vi "Measure.vi"(8 "error in":errorcluster, 10 "Measure Type":i32(ring) items=["Current", "High Current", "Low Current", "Max Current", "Min Current", "Power", "Voltage", "High Voltage", "Low Voltage", "Max Voltage", "Min Voltage", "A Hour", "W Hour", "Local Voltage", "Remote Voltage", "V/I/P/AHour/WHour", "Original Current", "Original Voltage", "UI interface Meter current", "UI Meter Voltage", "UI Meter power"], 11 "VISA resource name":refnum<visa-resource-name>) -> (0 "error out":errorcluster, 2 "Value":string, 3 "VISA resource name out":refnum<visa-resource-name>)   [LabVIEW 2015, in "IT-M3900C.lvlib"]
doc: "The MEASure subsystem command measures the output voltage or current.These commands will trigger the acquisition of additional data before the readings are returned.Perform the measurement by digitizing the instantaneous output voltage or current at the specified measurement time, storing the result in the buffer and calculating the value of the specified measurement type.\n\n<b>Measure Type</b>\n0:Current\n1:High Current\n2:Low Current\n3:Max Current\n4:Min Current\n5:Power\n6:Voltage\n7:High Voltage\n8:Low Voltage\n9:Max Voltage\n10:Min Voltage\n11:A Hour\n12:W Hour\n13:Local Voltage\n14:Remote Voltage\n15:V/I/P/AHour/WHour\n16:Original Current\n17:Original Voltage\n18:UI Meter current\n19:UI Meter voltage\n20:UI Meter power"
uses:
  <instrlib>/IT-M3900C/IT-M3900C.lvlib
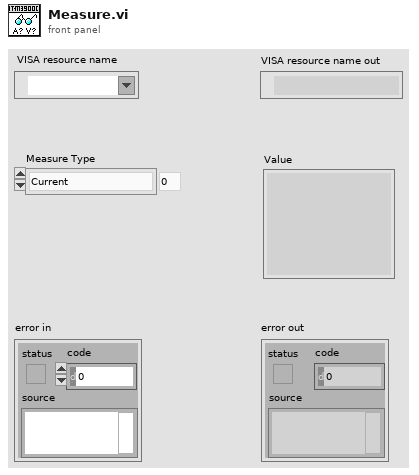
[diagram p1: front panel]
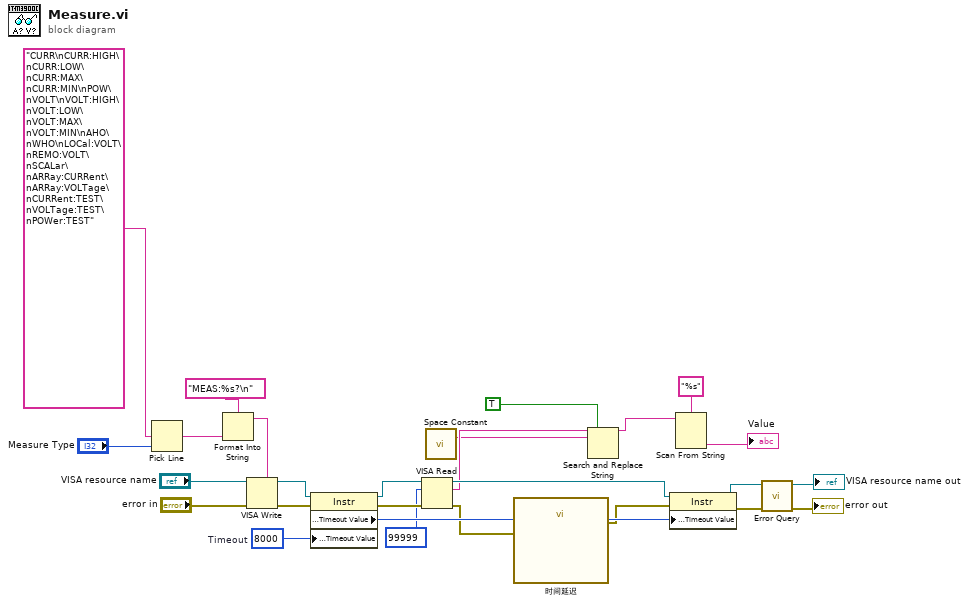
[diagram p0: block diagram]
diagram:
  w25 = u32 8000  # Timeout
  n1 = Pick Line(multi-line string="CURR\nCURR:HIGH\nCURR:LOW\nCURR:MAX\nCURR:MIN\nPOW\nVOLT\nVOLT:HIGH\nVOLT:LOW\nVOLT:MAX\nVOLT:MIN\nAHO\nWHO\nLOCal:VOLT\nREMO:VOLT\nSCALar\nARRay:CURRent\nARRay:VOLTage\nCURRent:TEST\nVOLTage:TEST\nPOWer:TEST", line index="Measure Type") -> (output string=w14:string)  [unwired: 1 in]
  n2 = Format Into String(format string="MEAS:%s?\n", w14) -> (resulting string=w17:string)  [unwired: 2 in, 1 out]
  n3 = VISA Write(VISA resource name="VISA resource name", write buffer=w17, error in (no error)="error in") -> (VISA resource name out=w27:refnum<visa-resource-name>, error out=w26:errorcluster)  [unwired: 1 out]
  n4 = property class="Instr"(reference=w27, error in=w26, "General Settings:Timeout Value"=w25) -> (reference out=w21:refnum<visa-resource-name>, error out=w22:errorcluster, "General Settings:Timeout Value"=w23:u32)
  n5 = VISA Read(VISA resource name=w21, byte count=99999, error in (no error)=w22) -> (VISA resource name out=w24:refnum<visa-resource-name>, read buffer=w5:string, error out=w2:errorcluster)  [unwired: 1 out]
  n6 = call <vilib>:"Space Constant.vi"() -> ("String"=w4:string)
  n7 = call "时间延迟"("error in (no error)"=w2) -> ("error out"=w1:errorcluster)  [unwired: 10 in]
  n8 = Search and Replace String(replace all?=TRUE ("替换全部？(F)"), input string=w5, search string=w4) -> (result string=w3:string)  [unwired: 5 in, 3 out]
  n9 = property class="Instr"(reference=w24, error in=w1, "General Settings:Timeout Value"=w23) -> (reference out=w7:refnum<visa-resource-name>, error out=w8:errorcluster)
  n10 = Scan From String(format string="%s", input string=w3) -> (output 1=→"Value":string)  [unwired: 3 in, 3 out]
  n11 = call <instrlib>:"Error Query.vi"("error in"=w8, "VISA resource name"=w7) -> ("error out"=→"error out":errorcluster, "VISA resource name out"=→"VISA resource name out":refnum<visa-resource-name>)  [unwired: 6 in, 2 out]
